vi "Init.vi"(10 "refs":T2, 11 "server queue":T3) -> (3 "RemoteConnection":refnum<class "RemoteConnection.lvclass">)   [LabVIEW 2013, in "RemoteConnection.lvclass"]
uses:
  RemoteConnection.lvclass
  message_queue.ctl
  Message/BaseMessage/BaseMessage.lvclass
  RemoteReferences.ctl
  response_event.ctl
  response.ctl
  driver_status.ctl
  RemoteConnection.lvclass/RemoteConnection.ctl
panel:
  out "response event":T1
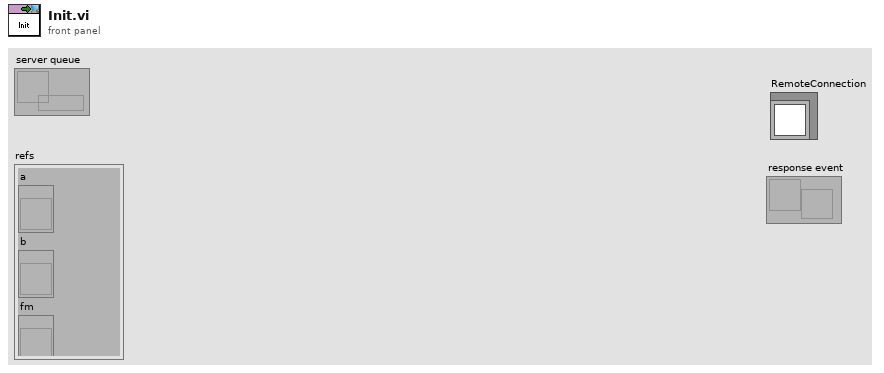
[diagram p1: front panel]
types:
  T1 = typedef "response_event.ctl" = refnum<user-event>
  T2 = typedef "RemoteConnection.lvclass/RemoteReferences.ctl" = cluster{"a":refnum<vi>, "b":refnum<vi>, "fm":refnum<vi>, "Output delay":refnum<vi>, "Output delay delta":refnum<vi>}
  T3 = typedef "message_queue.ctl" = refnum<queue>
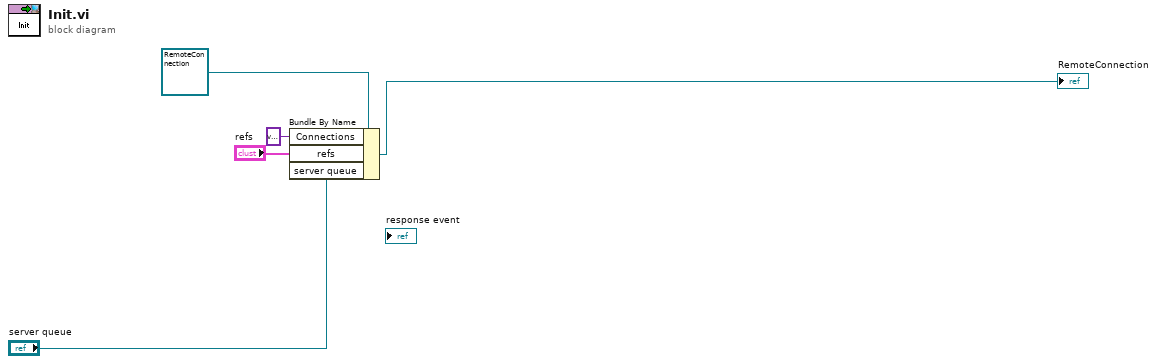
[diagram p0: block diagram]
diagram:
  n1 = Bundle By Name(cluster=refnum<class "RemoteConnection.lvclass"> refnum ("RemoteConnection"), "Connections"=variant, "refs"="refs", "server queue"="server queue") -> (→"RemoteConnection":refnum<class "RemoteConnection.lvclass">)
